vi "globalAntena.vi"() -> ()   [LabVIEW 2014]
panel:
  out "AntenaAltitud":dbl
  out "AntenaLongitud":dbl
  out "AntenaLatitud":dbl
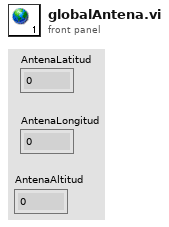
[diagram p1: front panel]
diagram:
